vi "Plant System.vi"(1 "Integrator?":bool, 2 "output saturation range":cluster{"output high":dbl, "output low":dbl}={"output high"=inf, "output low"=-inf}, 7 "Plant Input":dbl format="%.2f", 11 "dt (s)":dbl=-1.0 format="%.3f", 12 "reinitialize? (F)":bool, 13 "process parameters":T1={"static gain"=2.5, "lag (s)"=2.5, "deadtime (s)"=0.001, "load"=0.0, "deadband"=0.0, "sensor noise"=0.0, "initial PV"=5.0, "plant noise"=0.0} {"plant noise" format="%.3f"; "initial PV" format="%.3f"; "sensor noise" format="%.3f"; "lag (s)" format="%.3f"; "deadtime (s)" format="%.3f"; "deadband" format="%.3f"; "load" format="%.3f"; "static gain" format="%.3f"}) -> (8 "Plant Output":dbl format="%.2f")   [LabVIEW 2017]
doc: "Simulates a physical plant's response; for use with feedback control loops.\n\nAll scale factors are in percent. Lag time is in minutes. Process Deadtime is a true deadtime, measured as a multiple of the loop cycle time. NOTE: this deadtime is dependent upon the interval at which this VI is called. You can modify the algorithm used here to simulate almost any process.\n\nIf more than one plant needs to be simulated simultaneously, save multiple copies of this VI under different names."
uses:
  <vilib>/addons/control/pid/pid.llb/PID Lead-Lag (DBL).vi
  <vilib>/addons/control/pid/NI_PID_pid.lvlib
  <vilib>/addons/control/advanced/NI_AdvCtrl_nonlinear.lvlib
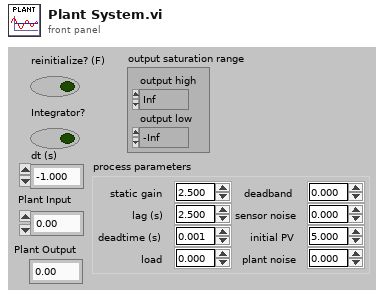
[diagram p1: front panel]
types:
  T1 = cluster{"static gain":dbl, "lag (s)":dbl, "deadtime (s)":dbl, "load":dbl, "deadband":dbl, "sensor noise":dbl, "initial PV":dbl, "plant noise":dbl}
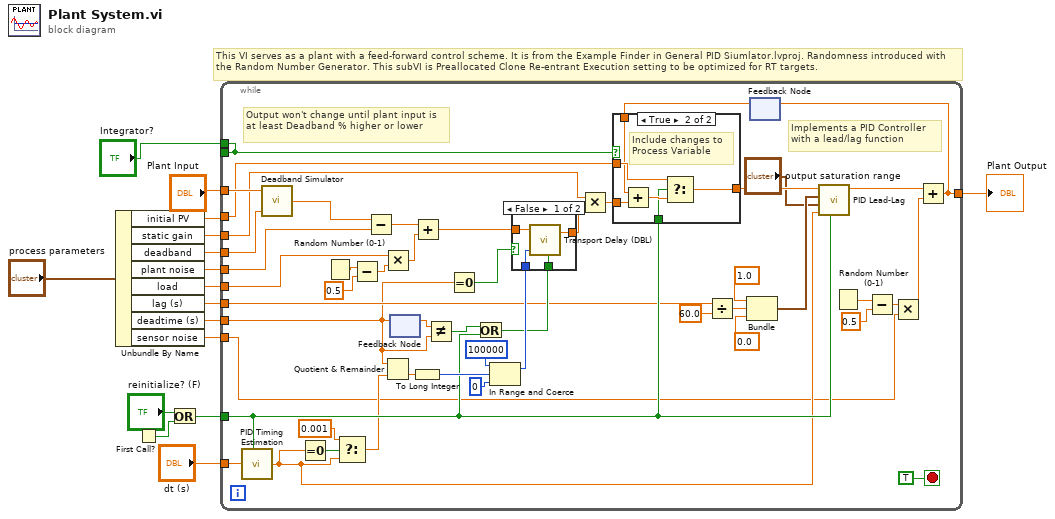
[diagram p0: block diagram]
diagram:
  # "This VI serves as a plant with a feed-forward control scheme. It is from the Example Finder in General PID Siumlator.lvproj. Randomness introduced with the Random Number Generator. This subVI is Preallocated Clone Re-entrant Execution setting to be optimized for RT targets."
  n1 = Unbundle By Name("process parameters") -> ("initial PV"=w3:dbl, "static gain"=w8:dbl, "deadband"=w7:dbl, "plant noise"=w4:dbl, "load"=w5:dbl, "lag (s)"=w10:dbl, "deadtime (s)"=w6:dbl, "sensor noise"=w2:dbl)
  n2 = First Call?() -> (First Call?: T/F=w15:bool)
  n3 = Or(x="reinitialize? (F)", y=w15) -> (x .or. y?=w14:bool)
  n4 = while {
    tunnel: w14 -> [w32]
    tunnel: "dt (s)" -> [w33]
    tunnel: [w49] -> w12
    tunnel: w5 -> [w18]
    tunnel: w10 -> [w23]
    tunnel: "Plant Input" -> [w30]
    tunnel: w8 -> [w29]
    tunnel: [w17] -> _
    tunnel: w7 -> [w24]
    tunnel: w6 -> [w21]
    tunnel: w4 -> [w19]
    tunnel: w3 -> [w22]
    tunnel: w2 -> [w20]
    tunnel: "Integrator?" -> [w17]
    stop <- TRUE stop-if-true
    # "Implements a PID Controller\nwith a lead/lag function"
    # "Output won't change until plant input is at least Deadband % higher or lower"
    n5 = call <vilib>:"PID Timing Estimation.vi"("Initialize?"=w32, "dt (s) in"=w33) -> ("dt (s) out"=w28:dbl)  [unwired: 7 in]
    n6 = call "Deadband Simulator.vi"("deadband (%)"=w24, "requested pos. (%)"=w30) -> ("actual pos. (%)"=w45:dbl)  [unwired: 1 in]
    n7 = Equal To 0?(x=w28) -> (x = 0?=w35:bool)
    n8 = Random Number (0-1)() -> (number: 0 to 1=w63:dbl)
    n9 = Select(t=0.001, s=w35, f=w28) -> (s? t:f=w26:dbl)
    n10 = Subtract(x=w63, y=0.5) -> (x-y=w31:dbl)
    n11 = Subtract(x=w45, y=w19) -> (x-y=w44:dbl)
    n12 = Multiply(x=w18, y=w31) -> (x*y=w65:dbl)
    n13 = Quotient & Remainder(x=w21, y=w26) -> (floor(x/y)=w51:dbl)  [unwired: 1 out]
    n14 = feedback-in #1(w21) -> ()
    n15 = feedback #1() -> (w41:dbl)  [unwired: 1 in]
    n16 = To Long Integer(number=w51) -> (32bit integer=w39:i32)
    n17 = Add(x=w44, y=w65) -> (x+y=w43:dbl)
    n18 = Not Equal?(x=w41, y=w21) -> (x != y?=w40:bool)
    n19 = Equal To 0?(x=w21) -> (x = 0?=w25:bool)
    n20 = Or(x=w40, y=w32) -> (x .or. y?=w27:bool)
    n21 = In Range and Coerce(upper limit=100000, x=w39, lower limit=0) -> (coerced(x)=w36:i32)  [unwired: 1 out]
    n22 = case shown="False" w25 {
      tunnel: [w69 w70] -> w50
      tunnel: w43 -> [w68 w70]
      tunnel: w36 -> [w67 _]
      tunnel: w27 -> [w66 _]
      frame False {
        n23 = call <vilib>:"Transport Delay (DBL).vi"("initialize"=w66, "delay"=w67, "input point"=w68) -> ("output point"=w69:dbl)  [unwired: 2 in]
      }
      frame True {
      }
    }
    n24 = Multiply(x=w29, y=w50) -> (x*y=w42:dbl)
    n25 = Divide(x=w23, y=60.0) -> (x/y=w47:dbl)
    n26 = Bundle(1.0, w47, 0.0) -> (w58:cluster{dbl, dbl, dbl})  [unwired: 1 in]
    n27 = feedback #2() -> (w57:dbl)  [unwired: 1 in]
    n28 = case shown="True" w17 {
      tunnel: w42 -> [w71 w77]
      tunnel: [w71 w75] -> w60
      tunnel: w22 -> [_ w74]
      tunnel: w57 -> [_ w73]
      tunnel: w32 -> [_ w72]
      frame False {
      }
      frame True {
        # "Include changes to Process Variable"
        n29 = Add(x=w73, y=w77) -> (x+y=w76:dbl)
        n30 = Select(t=w74, s=w72, f=w76) -> (s? t:f=w75:dbl)
      }
    }
    n31 = call-poly <vilib>:"PID Lead-Lag.vi"("reinitialize? (F)"=w32, "dt (s)"=w28, "output range"="output saturation range", "tuning parameters"=w58, "input"=w60) -> ("output"=w53:dbl)  [unwired: 3 in, 1 out]
    n32 = Random Number (0-1)() -> (number: 0 to 1=w56:dbl)
    n33 = Subtract(x=w56, y=0.5) -> (x-y=w55:dbl)
    n34 = Multiply(x=w55, y=w20) -> (x*y=w52:dbl)
    n35 = Add(x=w53, y=w52) -> (x+y=w49:dbl)
    n36 = feedback-in #2(w49) -> ()
  }
  "Plant Output" <- w12
